vi "ring_typedef.vi"(11 "State":T1 items=["s0", "s1"]) -> ()   [LabVIEW 2020]
uses:
  ring_typedef.ctl
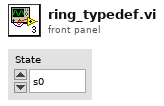
[diagram p1: front panel]
types:
  T1 = typedef "ring_typedef.ctl" = u16
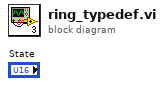
[diagram p0: block diagram]
diagram:
